vi "renameChannel.vi"() -> ()   [LabVIEW 2011, in "run.lvlib"]
uses:
  Hal/testing/run.lvlib
panel:
  out "error out":errorcluster
  in  "Replacement":string="MOT_Coil"
  in  "Channel":string="MOT coil"
  out "All Files in Dir":path[](array[path])
  in  "Path":path
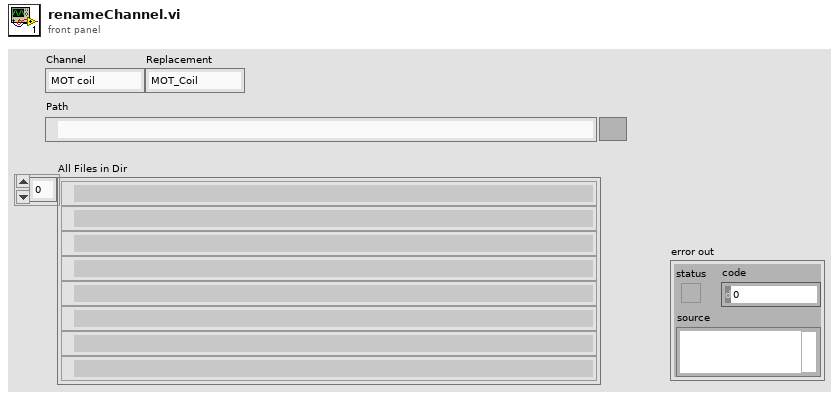
[diagram p1: front panel]
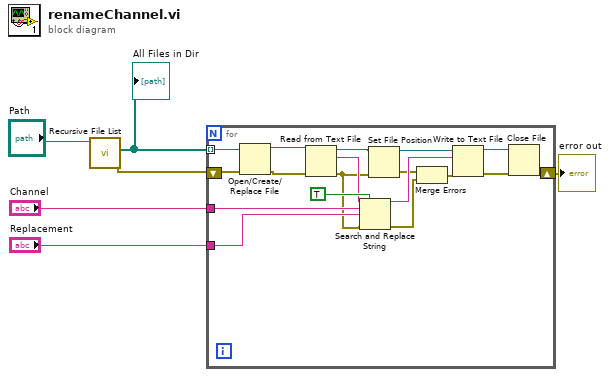
[diagram p0: block diagram]
diagram:
  n1 = call <vilib>:"Recursive File List.vi"("Folder Path"="Path") -> ("error out"=w4:errorcluster, "All Files in Dir"=w5:path[])  [unwired: 6 in, 3 out]
  "All Files in Dir" <- w5
  n2 = for {
    tunnel: w5 -> [w24] mode=indexing
    tunnel: "Channel" -> [w18]
    tunnel: "Replacement" -> [w17]
    shift-right: [w13] -> w1
    shift-left: w4 -> [w21]
    n3 = Open/Create/Replace File(file path (use dialog)=w24, error in=w21) -> (refnum out=w23:refnum<file>, error out=w22:errorcluster)  [unwired: 4 in, 1 out]
    n4 = Read from Text File(file (use dialog)=w23, error in=w22) -> (refnum out=w12:refnum<file>, text=w19:string, error out=w10:errorcluster)  [unwired: 2 in, 1 out]
    n5 = Search and Replace String(replace all?=TRUE ("replace all? (F)"), input string=w19, search string=w18, replace string=w17, error in=w10) -> (result string=w16:string, error out=w7:errorcluster)  [unwired: 3 in, 2 out]
    n6 = Set File Position(refnum=w12, error in=w10) -> (refnum out=w11:refnum<file>, error out=w8:errorcluster)  [unwired: 2 in]
    n7 = Merge Errors(w8, w7) -> (w9:errorcluster)
    n8 = Write to Text File(file (use dialog)=w11, text=w16, error in=w9) -> (refnum out=w14:refnum<file>, error out=w15:errorcluster)  [unwired: 1 in, 1 out]
    n9 = Close File(refnum=w14, error in=w15) -> (error out=w13:errorcluster)  [unwired: 1 out]
  }
  "error out" <- w1
